vi "Run_Core.vi"(0 "For Loop in":refnum<class "Structure Loop.lvclass">, 11 "error in (no error)":errorcluster) -> (4 "For Loop out":refnum<class "Structure Loop.lvclass">, 6 "Return":variant, 15 "error out":errorcluster)   [LabVIEW 2019, in "Structure Loop.lvclass"]
uses:
  Structure Loop.lvclass
  C:/Users/Patrick/Documents/GitHub/LabVIEW-Script-Language/source code/LSL components/functions/functionsbase/functionbase.lvclass
  functionsbase/functionbase.lvclass/functionbase.ctl
  Structure Loop.lvclass/Structure Loop.ctl
  functionsbase/properties/Read RT Variables.vi
  functionsbase/properties/Read Indent#.vi
  variables/RT Variables/RT Variables.lvclass
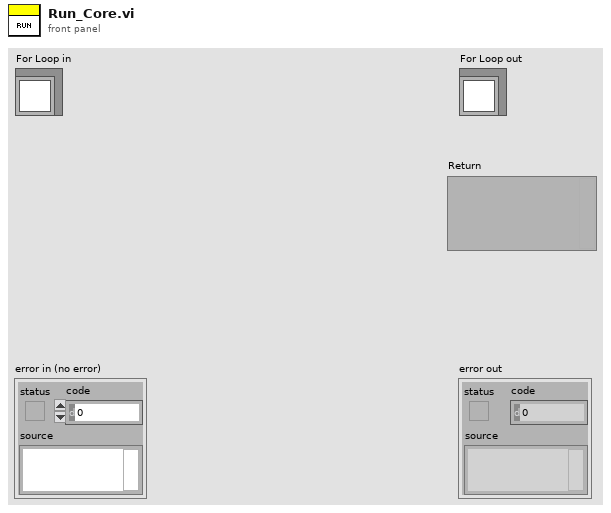
[diagram p1: front panel]
types:
  T1 = typedef "Structure Loop.lvclass/Function List.ctl" = enum16{"For Loop", "While Loop"}
  T2 = typedef "Datatype.ctl" = enum16{"Null", "Numeric", "String", "Bool", "Numeric 1D", "String 1D", "Bool 1D", "Numeric 2D", "String 2D", "Bool 2D", "Variant"}
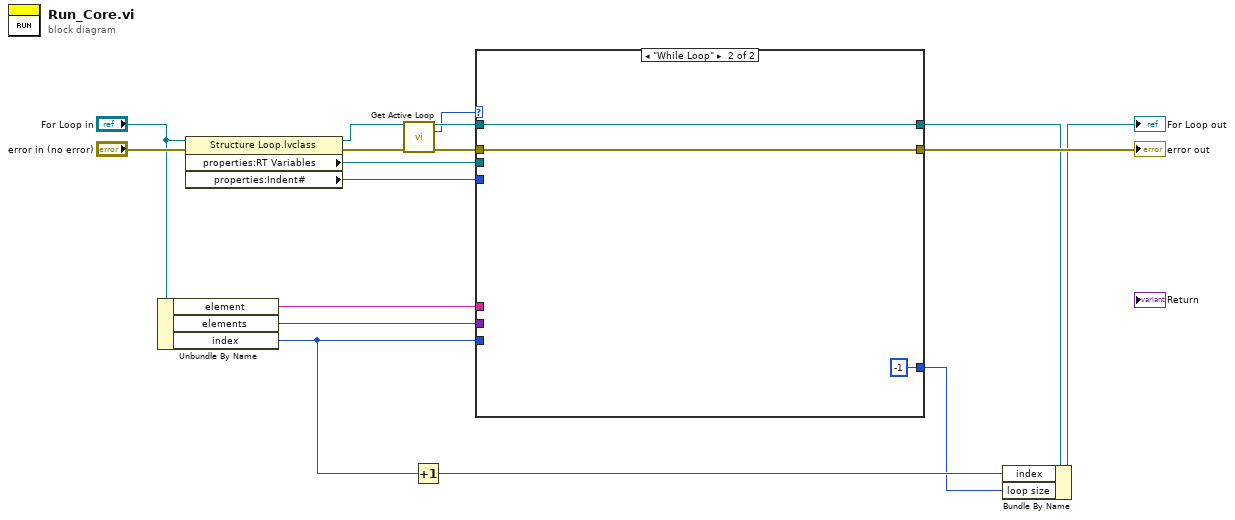
[diagram p0: block diagram]
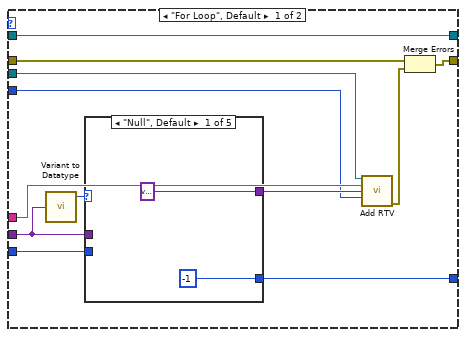
[diagram p2: hidden frame]
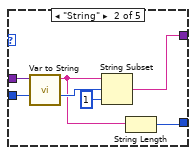
[diagram p3: hidden frame]
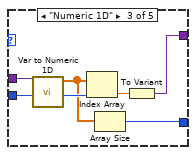
[diagram p4: hidden frame]
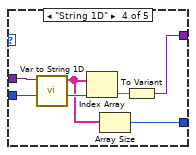
[diagram p5: hidden frame]
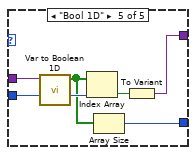
[diagram p6: hidden frame]
diagram:
  n1 = Unbundle By Name("For Loop in") -> ("element"=w7:string, "elements"=w8:variant, "index"=w3:i32)
  n2 = property class="Structure Loop.lvclass"(reference="For Loop in", error in="error in (no error)") -> (reference out=w10:refnum<class "Structure Loop.lvclass">, error out=w12:errorcluster, "properties:RT Variables"=w11:refnum<class "RT Variables.lvclass">, "properties:Indent#"=w6:i64)
  n3 = call "Get Active Loop.vi"("Structure Loop in"=w10, "error in (no error)"=w12) -> ("Structure Loop out"=w16:refnum<class "Structure Loop.lvclass">, "Function List"=w14:T1, "error out"=w15:errorcluster)  [unwired: 11 in]
  n4 = Increment(x=w3) -> (x+1=w2:i32)
  n5 = case shown="\"While Loop\"" w14 {
    tunnel: w16 -> [w29 w58]
    tunnel: [w29 w58] -> w5
    tunnel: w15 -> [w28 w57]
    tunnel: [w26 w57] -> w17
    tunnel: w11 -> [w27 _]
    tunnel: w8 -> [w22 _]
    tunnel: w7 -> [w24 _]
    tunnel: w3 -> [w21 _]
    tunnel: w6 -> [w19 _]
    tunnel: [w18 -1] -> w1
    frame "For Loop", Default {
      n6 = call "Variant to Datatype.vi"("Variant"=w22) -> ("Datatype"=w23:T2)  [unwired: 2 in, 2 out]
      n7 = case shown="\"Null\", Default" w23 {
        tunnel: w22 -> [_ w37 w43 w46 w52]
        tunnel: w21 -> [_ w36 w42 w49 w55]
        tunnel: [variant ("Variant") w34 w40 w47 w53] -> w20
        tunnel: [-1 w33 w38 w44 w50] -> w18
        frame "Null", Default {
        }
        frame "String" {
          n8 = call "Var to String.vi"("Variant"=w37) -> ("String"=w32:string)  [unwired: 10 in]
          n9 = String Subset(string=w32, offset (0)=w36, length (rest)=1 ("length (rest)")) -> (substring=w34:string)
          n10 = String Length(string=w32) -> (length=w33:i32)
        }
        frame "Numeric 1D" {
          n11 = call "Var to Numeric 1D.vi"("Variant"=w43) -> ("Numeric Array"=w39:dbl[])  [unwired: 10 in]
          n12 = Index Array(array=w39, index=w42) -> (element=w41:dbl)
          n13 = Array Size(array=w39) -> (size(s)=w38:i32)
          n14 = To Variant(anything=w41) -> (Variant=w40:variant)
        }
        frame "String 1D" {
          n15 = call "Var to String 1D.vi"("Variant"=w46) -> ("String 1D"=w45:string[])  [unwired: 10 in]
          n16 = Index Array(array=w45, index=w49) -> (element=w48:string)
          n17 = Array Size(array=w45) -> (size(s)=w44:i32)
          n18 = To Variant(anything=w48) -> (Variant=w47:variant)
        }
        frame "Bool 1D" {
          n19 = call "Var to Boolean 1D.vi"("Variant"=w52) -> ("Bool 1D"=w51:bool[])  [unwired: 10 in]
          n20 = Index Array(array=w51, index=w55) -> (element=w54:bool)
          n21 = Array Size(array=w51) -> (size(s)=w50:i32)
          n22 = To Variant(anything=w54) -> (Variant=w53:variant)
        }
      }
      n23 = call-dynamic "Add RTV.vi"("RT Variables in"=w27, "RTV name"=w24, "Data"=w20, "Scope"=w19) -> ("error out"=w25:errorcluster)  [unwired: 10 in, 1 out]
      n24 = Merge Errors(w28, w25) -> (w26:errorcluster)
    }
    frame "While Loop" {
    }
  }
  "error out" <- w17
  n25 = Bundle By Name(cluster=w5, "index"=w2, "loop size"=w1) -> (→"For Loop out":refnum<class "Structure Loop.lvclass">)
